vi "SerialNumber to DeviceName.vi"(8 "error in (no error)":errorcluster, 9 "NI2 Serial Number":dbl, 10 "NI1 Serial Number":dbl) -> (0 "error out":errorcluster, 1 "NI2 Device Name":tag, 2 "NI1 Device Name 2":tag)   [LabVIEW 2017]
uses:
  <resource>/objmgr/daqmx.rc
panel:
  in  "NI1 Serial Number 2":dbl
  in  "NI2 Serial Number 2":dbl
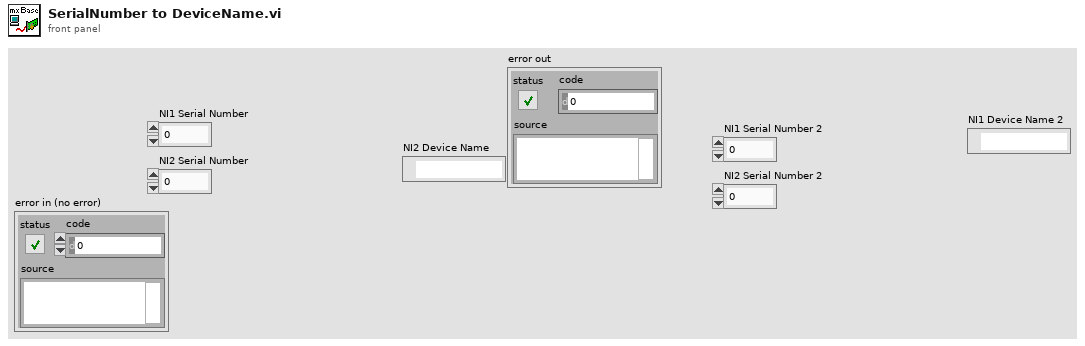
[diagram p1: front panel]
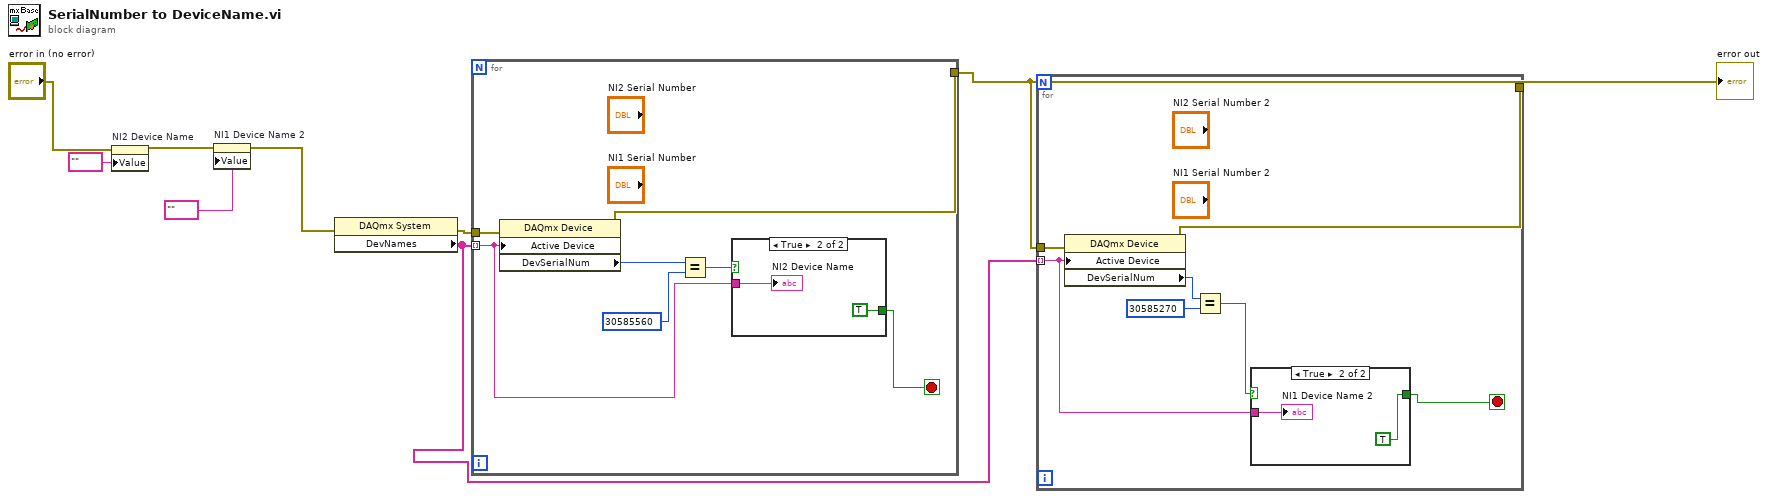
[diagram p0: block diagram]
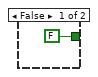
[diagram p2: hidden frame]
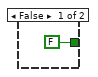
[diagram p3: hidden frame]
diagram:
  n1 = property on="NI2 Device Name" class="DAQmxName"(error in="error in (no error)", "Value"=tag "" ("NI2 Device Name")) -> (error out=w5:errorcluster)  [unwired: 1 in, 1 out]
  n2 = property on="NI1 Device Name 2" class="DAQmxName"(error in=w5, "Value"=tag "" ("NI1 Device Name 2")) -> (error out=w4:errorcluster)  [unwired: 1 in, 1 out]
  n3 = property class="DAQmx System"(error in=w4) -> (error out=w8:errorcluster, "DevNames"=w6:tag[])  [unwired: 1 in, 1 out]
  n4 = for {
    tunnel: w6 -> [w12] mode=indexing
    tunnel: w8 -> [w15]
    tunnel: [w14] -> w7
    stop <- w9 stop-if-true
    n5 = property class="DAQmx Device"(error in=w15, "Active Device"=w12) -> (error out=w14:errorcluster, "DevSerialNum"=w13:u32)  [unwired: 1 in, 1 out]
    n6 = Equal?(x=w13, y=30585560) -> (x = y?=w10:bool)
    n7 = case shown="True" w10 {
      tunnel: w12 -> [_ w18]
      tunnel: [FALSE TRUE] -> w9
      frame False {
      }
      frame True {
        "NI2 Device Name" <- w18
      }
    }
  }
  "error out" <- w7
  n8 = for {
    tunnel: w6 -> [w22] mode=indexing
    tunnel: w7 -> [w25]
    tunnel: [w24] -> _
    stop <- w19 stop-if-true
    n9 = property class="DAQmx Device"(error in=w25, "Active Device"=w22) -> (error out=w24:errorcluster, "DevSerialNum"=w23:u32)  [unwired: 1 in, 1 out]
    n10 = Equal?(x=w23, y=30585270) -> (x = y?=w20:bool)
    n11 = case shown="True" w20 {
      tunnel: w22 -> [_ w28]
      tunnel: [FALSE TRUE] -> w19
      frame False {
      }
      frame True {
        "NI1 Device Name 2" <- w28
      }
    }
  }
